vi "finalProject_interfaceLabVIEW.vi"(5 "stop":bool) -> (1 "Últimos Valores Registados:":string[](array[string]), 2 "Array":string[](array[string]), 3 "Waveform Chart":dynamicdata(graph)=[{"t0"=timestamp(3816698513.7637887 s since 1904-01-01), "dt"=1.0, "Y"=[0.0]}, {"t0"=timestamp(3816698513.7637887 s since 1904-01-01), "dt"=1.0, "Y"=[28.961962479327045]}])   [LabVIEW 2022 SP3]
uses:
  <vilib>/Instr/_visa.llb/VISA Flush IO Buffer Mask.ctl
  <vilib>/Platform/TimedLoop/XDataNode/timing_clust.ctl
  <vilib>/Platform/TimedLoop/XDataNode/nitl_modes.ctl
  <vilib>/Platform/TimedLoop/XDataNode/wakeup.ctl
  <vilib>/Utility/file.llb/Write Delimited Spreadsheet (string).vi
  <vilib>/Instr/_visa.llb/VISA Configure Serial Port (Instr).vi
  <vilib>/platform/TimedLoop/XDataNode/XDataNode.xnode
  <vilib>/Platform/TimedLoop/XDataNode/XDNodeRunTimeDep.lvlib
panel:
  out "Luminosidade (%)":sgl(slide) scale=0.0..100.0
  out "Histórico de Valores:":string[][](table)
  out "State":bool
  in  "Porta de Comunicação":refnum<visa-resource-name>="COM3-1"
  in  "Temp Setpoint (ºC)":sgl(knob)=25.0 scale=15.0..30.0 scale format="%#_2f"
  out "Temp Medida (ºC)":dbl(slide) scale=10.0..30.0
  out "Última Mensagem recebida do Arduino:":string
  in  "Diretoria de Dados Guardados:":path=path "C:/Users/celin/Documents/Alexandre Escola/Universidade/FEUP - Faculdade de Engenharia do Porto/1º Semestre/ASM - Aplicações de Sistemas Mecatrónicos/Arduino+LabView/Results.xls"
  # "Verde: Sistema Operacional\nAmarelo: Sistema Não Operacional"
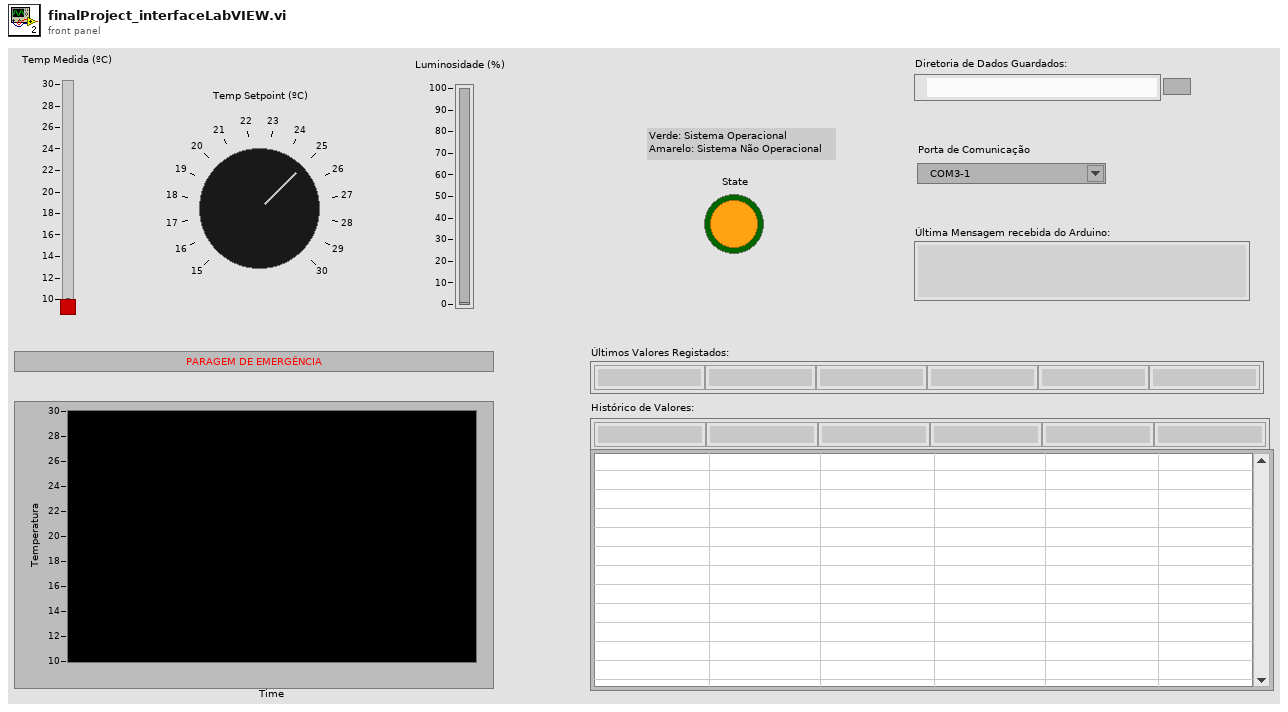
[diagram p1: front panel]
types:
  T1 = typedef "XDNodeRunTimeDep.lvlib/timing_clust.ctl" = cluster{"Expected End [f-1]":u64, "Actual End [f-1]":u64, "Finished Late? [f-1]":bool, "Expected End [i-1]":u64, "Actual End [i-1]":u64, "Finished Late? [i-1]":bool, "Expected Start [i]":u64, "Actual Start [i]":u64, "Expected Start [f]":u64, "Actual Start [f]":u64, "Source Name":string, "Structure Name":string, "Period":i64, "Deadline":i64, "Offset":i64, "Start":i64, "Priority":i32, "Timeout":i32, "Mode":T2, "Wakeup Reason":T3, "Error":errorcluster, "Source Type":string, "Secondary Source Type":string, "Global End Time":u64, "Global Start Time":u64, "Frame Duration":u64, "Iteration Duration":u64, "Assigned CPU":i32, "I/O Scan Engine Mode":u32}
  T2 = typedef "XDNodeRunTimeDep.lvlib/nitl_modes.ctl" = enum32{"No Change", "Process missed periods, maintain original phase", "Discard missed periods, maintain original phase", "Process missed periods, ignore original phase", "Discard missed periods, ignore original phase"}
  T3 = typedef "XDNodeRunTimeDep.lvlib/wakeup.ctl" = enum32{"Normal", "Aborted", "Asynchronous wakeup", "Timing source error", "Timed loop error", "Timeout"}
  T4 = typedef "VISA Flush IO Buffer Mask.ctl" = u16
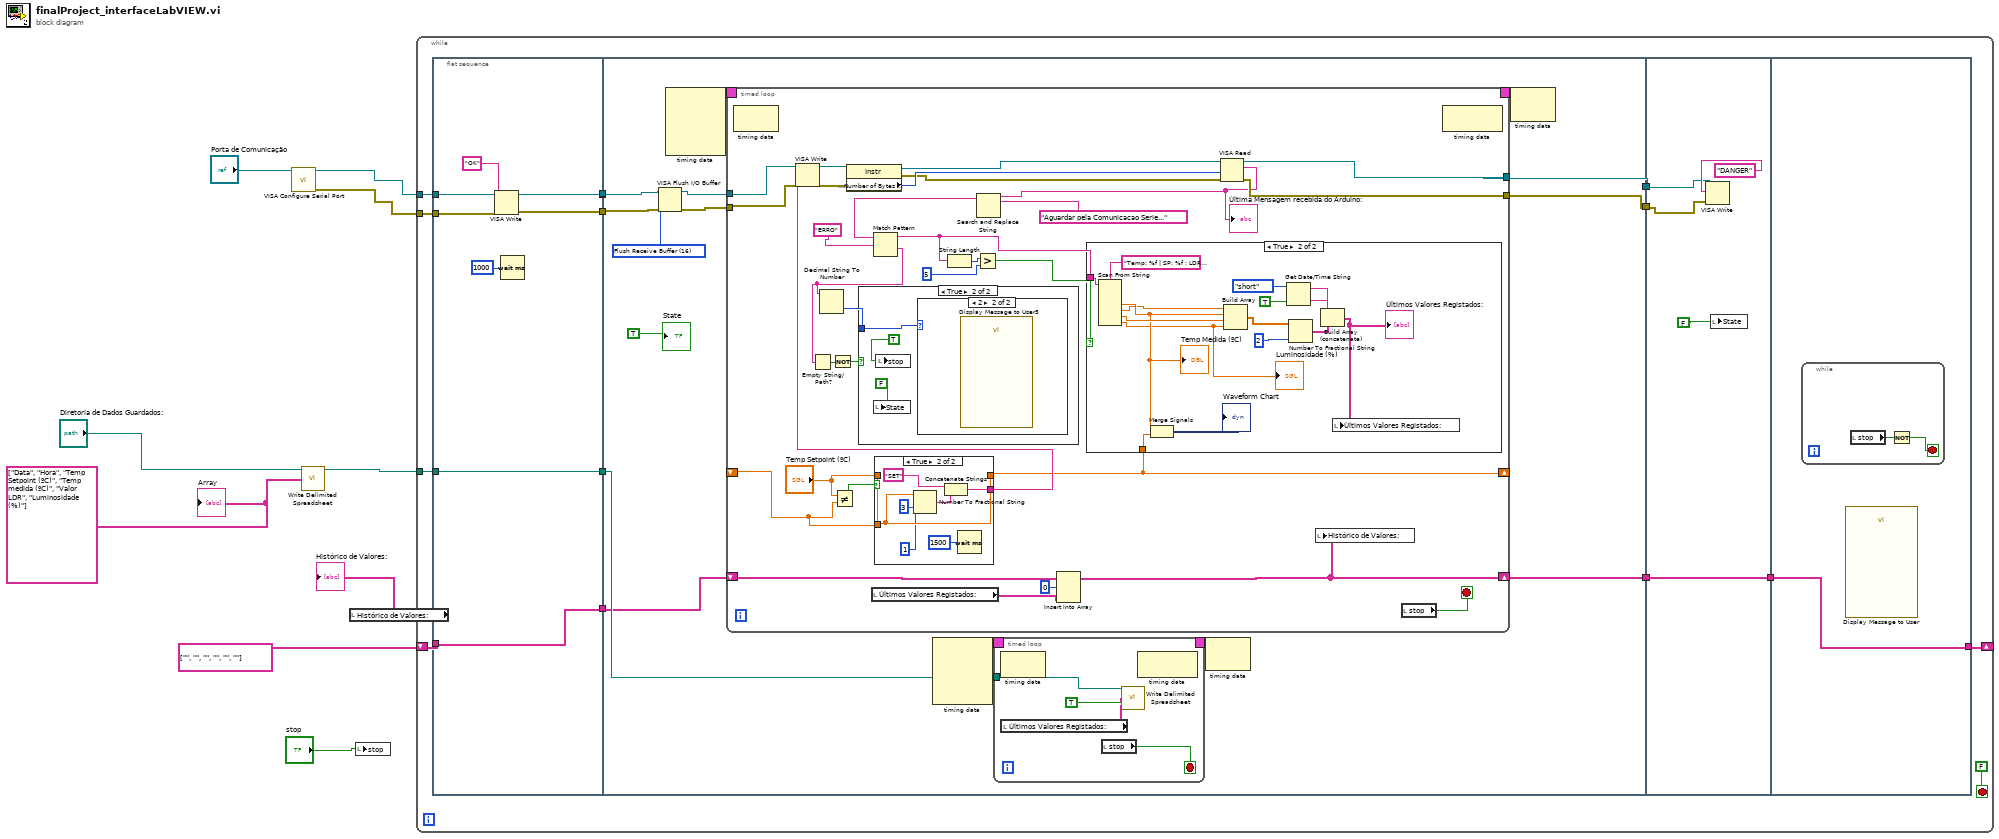
[diagram p0: block diagram]
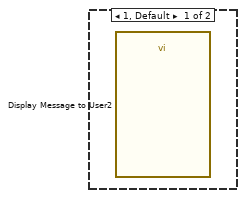
[diagram p3: hidden frame]
diagram:
  w7 = string[] ["Data", "Hora", "Temp Setpoint (ºC)", "Temp medida (ºC)", "Valor LDR", "Luminosidade (%)"]
  n1 = call-poly "VISA Configure Serial Port"("VISA resource name"="Porta de Comunicação") -> ("VISA resource name out"=w3:refnum<visa-resource-name>, "error out"=w4:errorcluster)  [unwired: 13 in]
  n2 = call-poly <vilib>:"Write Delimited Spreadsheet.vi"("file path (dialog if empty)"="Diretoria de Dados Guardados:", "1D data"=w7) -> ("new file path (Not A Path if cancelled)"=w6:path)  [unwired: 12 in, 1 out]
  n3 = local read "Histórico de Valores:"() -> (→"Histórico de Valores:":string[][])
  n4 = local write "stop"("stop") -> ()
  n5 = while {
    tunnel: w6 -> [w18]
    tunnel: w4 -> [w15]
    tunnel: w3 -> [w14]
    shift-right: [w11] -> _
    shift-left: string[][] [["", "", "", "", "", ""]] -> [w10]
    stop <- FALSE stop-if-true
    n6 = flat-sequence {
      tunnel: [w31] -> w24
      tunnel: [w30] -> w23
      tunnel: [w29] -> w22
      tunnel: [w28] -> w21
      tunnel: w14 -> [w31]
      tunnel: w15 -> [w30]
      tunnel: w18 -> [w29]
      tunnel: [w25] -> w16
      tunnel: w10 -> [w25]
      tunnel: w24 -> [_]
      tunnel: w23 -> [w34]
      tunnel: w22 -> [w40]
      tunnel: [w46] -> w20
      tunnel: [w45] -> w19
      tunnel: w21 -> [w39]
      tunnel: w16 -> [w36]
      tunnel: [w32] -> w13
      tunnel: w20 -> [w119]
      tunnel: w19 -> [w120]
      tunnel: w13 -> [w117]
      tunnel: [w117] -> w12
      tunnel: w12 -> [w122]
      tunnel: [w122] -> w11
      frame #0 {
        n7 = VISA Write(VISA resource name=w31, write buffer="OK", error in (no error)=w30) -> (VISA resource name out=w28:refnum<visa-resource-name>)  [unwired: 2 out]
        n8 = Wait (ms)(milliseconds to wait=u32 1000) -> ()  [unwired: 1 out]
      }
      frame #1 {
        w37 = T4 16 items=["Flush Receive Buffer"=16, "Write Transmit Buffer to Device"=32, "Flush Receive Buffer (No I/O)"=64, "Flush Transmit Buffer"=128] ("Mask")
        n9 = VISA Flush I/O Buffer(VISA resource name=w39, mask (16)=w37, error in (no error)=w34) -> (VISA resource name out=w38:refnum<visa-resource-name>, error out=w35:errorcluster)
        n10 = node-c288() -> (w44:T1)  [unwired: 4 in]
        n11 = timed-loop {
          tunnel: [w85] -> w45
          tunnel: [w84] -> w46
          shift-right: [w55] -> _
          shift-left: _ -> [w75]
          timing: w44 -> [_]
          timing-out: [_] -> w43
          tunnel: w38 -> [w74]
          shift-right: [w56] -> w32
          shift-left: w36 -> [w72]
          tunnel: w35 -> [w62]
          stop <- w73 stop-if-true
          n12 = node-c288() -> ()  [unwired: 1 in, 1 out]
          n13 = Not Equal?(x="Temp Setpoint (ºC)", y=w75) -> (x != y?=w77:bool)
          n14 = local read "Últimos Valores Registados:"() -> (w71:string[])
          n15 = case shown="True" w77 {
            tunnel: [w107 w112] -> w55
            tunnel: "Temp Setpoint (ºC)" -> [_ w112]
            tunnel: [_ w110] -> w80
            tunnel: w75 -> [w107 _]
            frame False {
            }
            frame True {
              n16 = Number To Fractional String(number=w112, width (-)=i16 3, precision (6)=i16 1 ("width (-)")) -> (F-format string=w113:string)  [unwired: 1 in]
              n17 = Concatenate Strings("SET", w113) -> (w110:string)
              n18 = Wait (ms)(milliseconds to wait=u32 1500) -> ()  [unwired: 1 out]
            }
          }
          n19 = VISA Write(VISA resource name=w74, write buffer=w80, error in (no error)=w62) -> (VISA resource name out=w79:refnum<visa-resource-name>, error out=w78:errorcluster)  [unwired: 1 out]
          n20 = property class="Instr"(reference=w79, error in=w78) -> (reference out=w83:refnum<visa-resource-name>, error out=w81:errorcluster, "Serial Settings:Number of Bytes at Serial Port"=w82:u32)
          n21 = Insert Into Array(array=w72, index (row)=0, new element=w71) -> (w56:string[][])  [unwired: 1 in]
          n22 = VISA Read(VISA resource name=w83, byte count=w82, error in (no error)=w81) -> (VISA resource name out=w85:refnum<visa-resource-name>, read buffer=w66:string, error out=w84:errorcluster)  [unwired: 1 out]
          "Última Mensagem recebida do Arduino:" <- w66
          n23 = Search and Replace String(input string=w66, search string="Aguardar pela Comunicacao Serie...") -> (result string=w65:string)  [unwired: 6 in, 3 out]
          n24 = Match Pattern(string=w65, regular expression="ERRO") -> (before substring=w69:string, after substring=w57:string)  [unwired: 1 in, 2 out]
          n25 = Empty String/Path?(string/path=w57) -> (empty?=w60:bool)
          n26 = Decimal String To Number(string=w57) -> (number=w58:i32)  [unwired: 2 in, 1 out]
          n27 = Not(x=w60) -> (.not. x?=w59:bool)
          n28 = case shown="True" w59 {
            tunnel: w58 -> [_ w88]
            frame False {
            }
            frame True {
              n29 = local write "State"(FALSE ("Boolean")) -> ()
              n30 = local write "stop"(TRUE ("stop")) -> ()
              n31 = case shown="2" w88 {
                frame 1, Default {
                  n32 = call "Display Message to User2"() -> ()  [unwired: 10 in, 2 out]
                }
                frame 2 {
                  n33 = call "Display Message to User3"() -> ()  [unwired: 10 in, 2 out]
                }
              }
            }
          }
          n34 = String Length(string=w69) -> (length=w68:i32)
          n35 = Greater?(x=w68, y=5) -> (0:w67:bool)
          n36 = case shown="True" w67 {
            tunnel: w69 -> [_ w92]
            tunnel: w55 -> [_ w89]
            frame False {
            }
            frame True {
              n37 = Scan From String(format string="Temp: %f | SP: %f ; LDR Value: %f | Light Level: %f%", input string=w92) -> (output 1=w96:dbl, output 2=w90:dbl, output 3=w103:dbl, output 4=w91:sgl)  [unwired: 6 in, 3 out]
              "Temp Medida (ºC)" <- w96
              "Luminosidade (%)" <- w91
              n38 = Merge Signals(w96, w89) -> (→"Waveform Chart":dynamicdata)
              n39 = Build Array(w90, w96, w103, w91) -> (w95:dbl[])
              n40 = Get Date/Time String(date format (0)=enum16{"short", "long", "abbreviated"}."short", want seconds? (F)=TRUE) -> (date string=w100:string, time string=w99:string)  [unwired: 1 in]
              n41 = Number To Fractional String(number=w95, precision (6)=i16 2) -> (F-format string=w101:string[])  [unwired: 2 in]
              n42 = Build Array (concatenate)(w100, w99, w101) -> (w94:string[])
              "Últimos Valores Registados:" <- w94
              n43 = local write "Últimos Valores Registados:"(w94) -> ()
            }
          }
          n44 = local write "Histórico de Valores:"(w56) -> ()
          n45 = local read "stop"() -> (w73:bool)
          n46 = node-c288() -> ()  [unwired: 1 in, 1 out]
        }
        n47 = node-c288() -> (w42:T1)  [unwired: 4 in]
        n48 = timed-loop {
          timing: w42 -> [_]
          timing-out: [_] -> w41
          tunnel: w40 -> [w50]
          stop <- w48 stop-if-true
          n49 = node-c288() -> ()  [unwired: 1 in, 1 out]
          n50 = local read "Últimos Valores Registados:"() -> (w47:string[])
          n51 = local read "stop"() -> (w48:bool)
          n52 = call-poly <vilib>:"Write Delimited Spreadsheet.vi"("file path (dialog if empty)"=w50, "1D data"=w47, "append to file? (new file:F)"=TRUE) -> ()  [unwired: 11 in, 2 out]
          n53 = node-c288() -> ()  [unwired: 1 in, 1 out]
        }
        n54 = node-c288(w41) -> ()  [unwired: 1 out]
        n55 = node-c288(w43) -> ()  [unwired: 1 out]
        "State" <- TRUE ("Boolean")
      }
      frame #2 {
        n56 = VISA Write(VISA resource name=w120, write buffer="DANGER", error in (no error)=w119) -> ()  [unwired: 3 out]
        n57 = local write "State"(FALSE) -> ()
      }
      frame #3 {
        n58 = while {
          stop <- w123 stop-if-true
          n59 = local read "stop"() -> (w124:bool)
          n60 = Not(x=w124) -> (.not. x?=w123:bool)
        }
        n61 = call "Display Message to User"() -> ()  [unwired: 10 in, 2 out]
      }
    }
  }
  "Array" <- w7
